vi "GetLineMovement.vi"(4 "Sign":dbl, 5 "Total Angle [rad]":dbl, 6 "Motion Time per Line [s]":dbl, 7 "Line Length [mm]":dbl, 8 "Relative Line\nSeparations [mm]":dbl[](array[numeric]), 9 "Start Position":dbl[](array[numeric])) -> (0 "Line Motion":T2, 1 "Motion Speed [mm/s]":T1, 2 "Move across Line [mm]":dbl[](array[numeric]), 3 "Move to Start of Line [mm]":dbl[](array[numeric]))   [LabVIEW 2016]
panel:
  in  "Default Axis Speeds":T1={"X [mm/s]"=25.0, "Y [mm/s]"=25.0, "Z [mm/s]"=25.0}
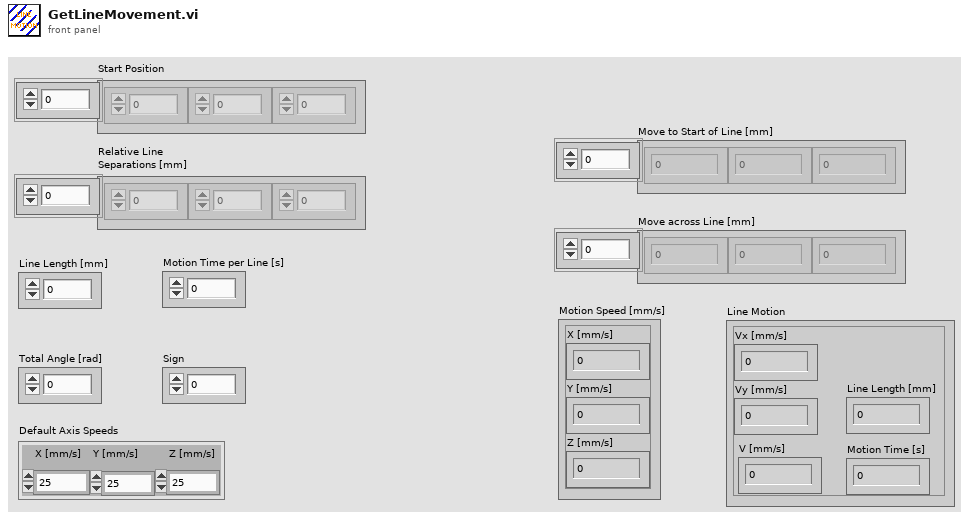
[diagram p1: front panel]
types:
  T1 = cluster{"X [mm/s]":dbl, "Y [mm/s]":dbl, "Z [mm/s]":dbl}
  T2 = cluster{"Vx [mm/s]":dbl, "Vy [mm/s]":dbl, "Numeric Control":dbl, "Numeric Control":dbl, "Line Length [mm]":dbl}
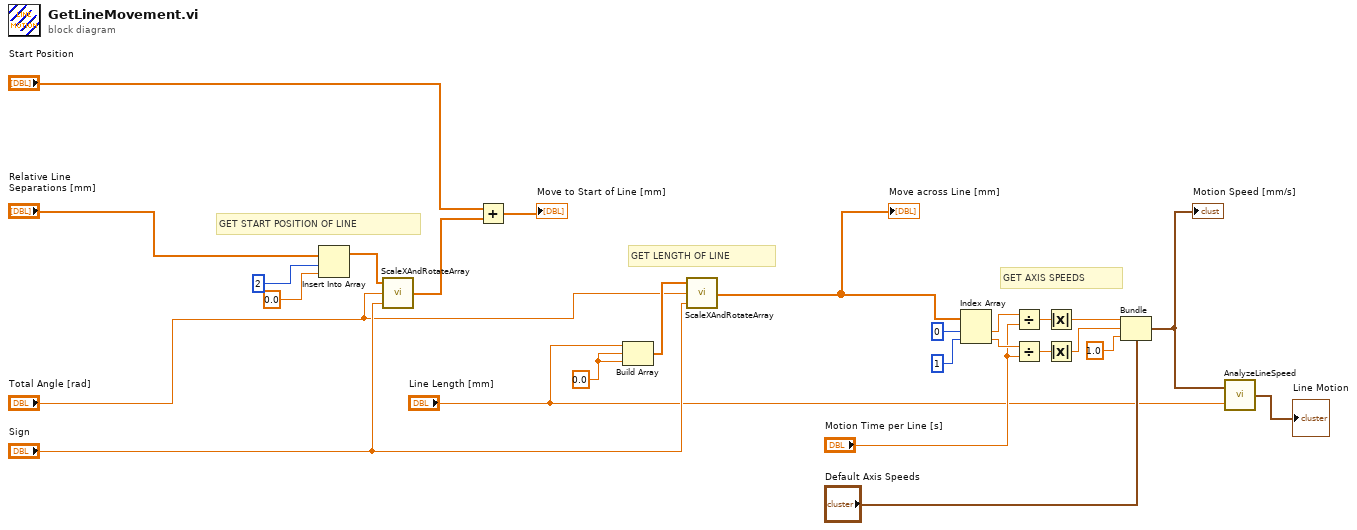
[diagram p0: block diagram]
diagram:
  w16 = 0.0 ("element")
  # "GET START POSITION OF LINE"
  # "GET LENGTH OF LINE"
  # "GET AXIS SPEEDS"
  n1 = Insert Into Array(array="Relative Line\nSeparations [mm]", index=2, new element=0.0 ("new element/subarray")) -> (w12:dbl[])
  n2 = call "ScaleXAndRotateArray.vi"("Scale"="Sign", "Angle"="Total Angle [rad]", "X, Y, Z Input"=w12) -> ("c * X', Y', Z Output"=w11:dbl[])
  n3 = Add(x="Start Position", y=w11) -> (x+y=→"Move to Start of Line [mm]":dbl[])
  n4 = Build Array("Line Length [mm]", w16, w16) -> (w15:dbl[])
  n5 = call "ScaleXAndRotateArray.vi"("Scale"="Sign", "Angle"="Total Angle [rad]", "X, Y, Z Input"=w15) -> ("c * X', Y', Z Output"=w1:dbl[])
  "Move across Line [mm]" <- w1
  n6 = Index Array(array=w1, index #1=0 ("index"), index #2=1 ("index")) -> (element #1=w22:dbl, element #2=w21:dbl)
  n7 = Divide(x=w22, y="Motion Time per Line [s]") -> (x/y=w20:dbl)
  n8 = Divide(x=w21, y="Motion Time per Line [s]") -> (x/y=w19:dbl)
  n9 = Absolute Value(x=w20) -> (abs(x)=w18:dbl)
  n10 = Absolute Value(x=w19) -> (abs(x)=w17:dbl)
  n11 = Bundle(cluster="Default Axis Speeds", "X [mm/s]"=w18, "Y [mm/s]"=w17, "Z [mm/s]"=1.0) -> (w7:T1)
  "Motion Speed [mm/s]" <- w7
  n12 = call "AnalyzeLineSpeed.vi"("Line Length [mm]"="Line Length [mm]", "Line Speeds [mm/s]"=w7) -> ("Output"=→"Line Motion":T2)
